vi "init.vi"(8 "error in (no error)":errorcluster, 11 "Logger in":refnum<class "TestDataLog.lvclass">) -> (0 "error out":errorcluster, 3 "Logger out":refnum<class "TestDataLog.lvclass">)   [LabVIEW 2013, in "TestDataLog.lvclass"]
uses:
  TestDataLog.lvclass
  Configuration/SystemController.ctl
  Configuration/PIDGains.ctl
  <userlib>/Common/Log/Config/Log.ctl
  Configuration/TestParameters.ctl
  Configuration/CycleProfileConfig.ctl
  TestDataLog.lvclass/TestDataLog.ctl
  <userlib>/Common/Log/Log/Log.lvclass/Log.ctl
  ConfigurationThisComponent/ConfigurationThisComponent.lvclass
  <userlib>/Common/Log/Log/Log.lvclass
  <userlib>/Common/Log/Log.lvlib
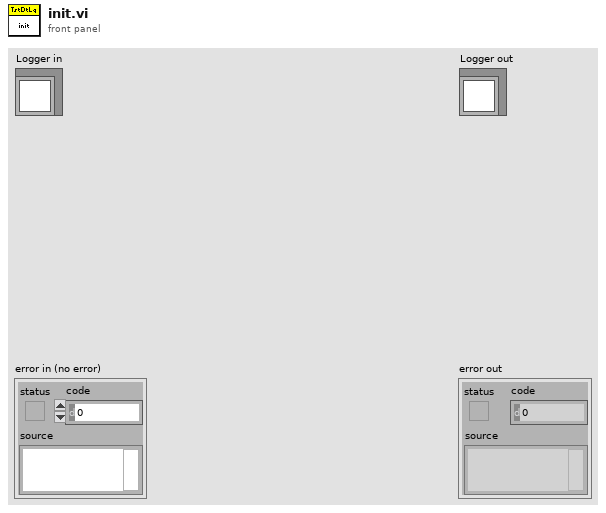
[diagram p1: front panel]
types:
  T1 = typedef "TestParameters.ctl" = cluster{"Number of cycles for complete test":u32, "Cycle profile":T2}
  T2 = typedef "CycleProfileConfig.ctl" = cluster{"Force Setpoint":dbl[unit][], "Pause After":dbl[unit][]}
  T3 = typedef "Log.lvlib/Log.ctl" = cluster{"Log Directory":path, "Log Filename Base":string, "Max records per file":u32, "Comment":string}
  T4 = typedef "SystemController.ctl" = cluster{"PID Gains":T5, "Force Error In Range Limit":dbl[unit]}
  T5 = typedef "PIDGains.ctl" = cluster{"Proportional Gain (Kc)":dbl, "Integral Time (Ti, min)":dbl, "Derivative Time (Td, min)":dbl}
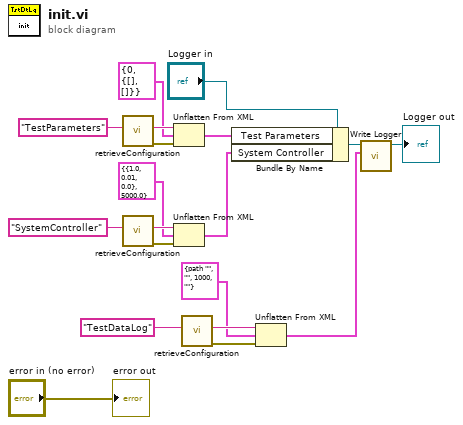
[diagram p0: block diagram]
diagram:
  n1 = call "retrieveConfiguration.vi"("configName"="TestParameters") -> ("error out"=w5:errorcluster, "xmlConfig"=w4:string)  [unwired: 8 in, 1 out]
  n2 = call "retrieveConfiguration.vi"("configName"="SystemController") -> ("error out"=w17:errorcluster, "xmlConfig"=w16:string)  [unwired: 8 in, 1 out]
  n3 = Unflatten From XML(xml string=w4, type=T1 {"Number of cycles for complete test"=0, "Cycle profile"={"Force Setpoint"=[], "Pause After"=[]}} ("Test Parameters"), error in (no error)=w5) -> (value=w2:T1)  [unwired: 1 out]
  n4 = Unflatten From XML(xml string=w16, type=T4 {"PID Gains"={"Proportional Gain (Kc)"=1.0, "Integral Time (Ti, min)"=0.01, "Derivative Time (Td, min)"=0.0}, "Force Error In Range Limit"=5000.0} ("System Controller"), error in (no error)=w17) -> (value=w14:T4)  [unwired: 1 out]
  n5 = call "retrieveConfiguration.vi"("configName"="TestDataLog") -> ("error out"=w11:errorcluster, "xmlConfig"=w12:string)  [unwired: 8 in, 1 out]
  n6 = Bundle By Name(cluster="Logger in", "Test Parameters"=w2, "System Controller"=w14) -> (w9:refnum<class "TestDataLog.lvclass">)
  n7 = Unflatten From XML(xml string=w12, type=T3 {"Log Directory"=path "", "Log Filename Base"="", "Max records per file"=1000, "Comment"=""} ("Logger"), error in (no error)=w11) -> (value=w7:T3)  [unwired: 1 out]
  n8 = call <userlib>:"Write Logger.vi"("Logger"=w7, "Logger in"=w9) -> ("Logger out"=→"Logger out":refnum<class "TestDataLog.lvclass">)  [unwired: 9 in]
  "error out" <- "error in (no error)"
